vi "Drive Motor Joysticks.vi"(8 "Boost?":bool, 9 "Turn":dbl, 10 "Throttle":dbl, 11 "Auto-Align?":bool) -> (2 "Teleop Drive command":T1)   [LabVIEW 2019]
uses:
  Drive Command Typedef.ctl
  Drive Mode Typedef.ctl
  <vilib>/Rock Robotics/Network Tables/NT Read Number.vi
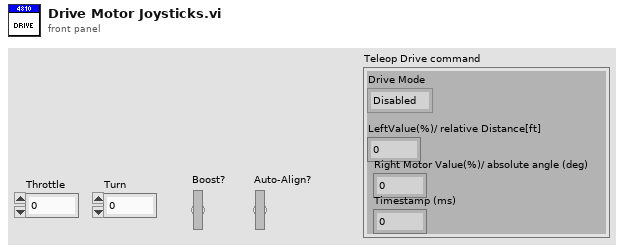
[diagram p1: front panel]
types:
  T1 = typedef "Drive Command Typedef.ctl" = cluster{"Drive Mode":T2, "LeftValue(%)/ relative Distance[ft]":dbl, "Right Motor Value(%)/ absolute angle (deg)":dbl, "Timestamp (ms)":dbl}
  T2 = typedef "Drive Mode Typedef.ctl" = enum16{"Disabled", "Auto-align", "Drive Distance", "Turn to angle", "Driver", "Driver Velocity Control"}
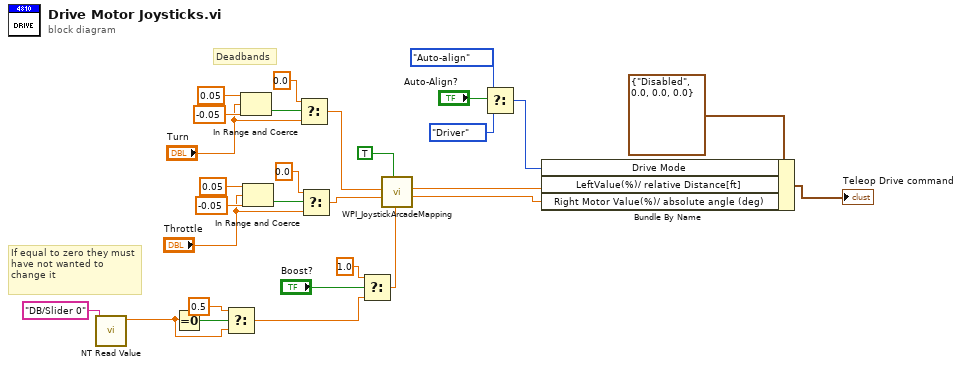
[diagram p0: block diagram]
diagram:
  # "If equal to zero they must have not wanted to change it"
  # "Deadbands"
  n1 = call-poly <vilib>:"NT Read Value.vi"("Name"="DB/Slider 0") -> ("Numeric"=w2:dbl)  [unwired: 9 in, 1 out]
  n2 = Equal To 0?(x=w2) -> (x = 0?=w4:bool)
  n3 = Select(t=0.5 ("f"), s=w4, f=w2) -> (s? t:f=w1:dbl)
  n4 = In Range and Coerce(upper limit=0.05 ("t"), x="Turn", lower limit=-0.05 ("t")) -> (In Range?=w17:bool)  [unwired: 1 out]
  n5 = In Range and Coerce(upper limit=0.05 ("t"), x="Throttle", lower limit=-0.05 ("t")) -> (In Range?=w11:bool)  [unwired: 1 out]
  n6 = Select(t=0.0, s=w17, f="Turn") -> (s? t:f=w12:dbl)
  n7 = Select(t=0.0, s=w11, f="Throttle") -> (s? t:f=w6:dbl)
  n8 = Select(t=1.0, s="Boost?", f=w1) -> (s? t:f=w26:dbl)
  n9 = call <vilib>:"WPI_JoystickArcadeMapping.vi"("Max Output"=w26, "Square Inputs"=TRUE, "Y axis value"=w6, "X axis value"=w12) -> ("Right Motor Value"=w24:dbl, "Left Motor Value"=w25:dbl)  [unwired: 6 in]
  n10 = Select(t=Drive_Mode_Typedef."Auto-align" ("Drive Mode"), s="Auto-Align?", f=Drive_Mode_Typedef."Driver" ("Drive Mode")) -> (s? t:f=w21:T2)
  n11 = Bundle By Name(cluster=T1 {"Drive Mode"=enum."Disabled", "LeftValue(%)/ relative Distance[ft]"=0.0, "Right Motor Value(%)/ absolute angle (deg)"=0.0, "Timestamp (ms)"=0.0} ("Drive Command"), "Drive Mode"=w21, "LeftValue(%)/ relative Distance[ft]"=w25, "Right Motor Value(%)/ absolute angle (deg)"=w24) -> (→"Teleop Drive command":T1)
